vi "Delay.vi"(2 "error in (no error)":errorcluster, 3 "Delay Time (s)":dbl=1.0) -> (0 "error out":errorcluster)   [LabVIEW 2019]
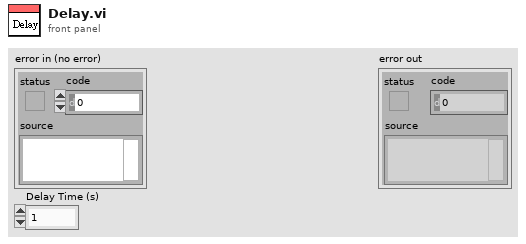
[diagram p1: front panel]
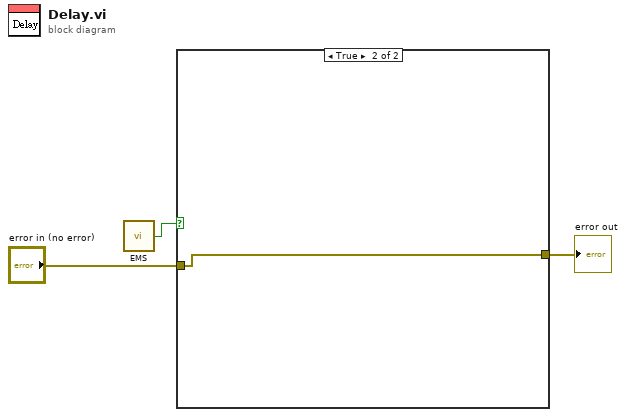
[diagram p0: block diagram]
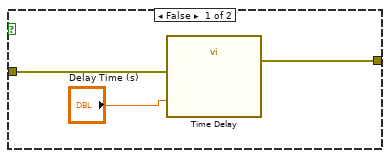
[diagram p2: hidden frame]
diagram:
  n1 = call "EMS.vi"() -> ("A/DIO4 (Pin 19)"=w1:bool)
  n2 = case shown="True" w1 {
    tunnel: "error in (no error)" -> [w6 w7]
    tunnel: [w4 w7] -> w2
    frame False {
      n3 = call "Time Delay"("error in (no error)"=w6, "Delay Time (s)"="Delay Time (s)") -> ("error out"=w4:errorcluster)  [unwired: 9 in]
    }
    frame True {
    }
  }
  "error out" <- w2
